vi "Table_AddNewChannelToChannelList.vi"(10 "Channel":T1, 11 "Channels":T1[](array[typedef])) -> (3 "Channels Out":T1[](array[typedef]))   [LabVIEW 2012, in "TableSupportLib.lvlib"]
uses:
  TableSupportLib.lvlib
  Table_ChannelInfoCluster.ctl
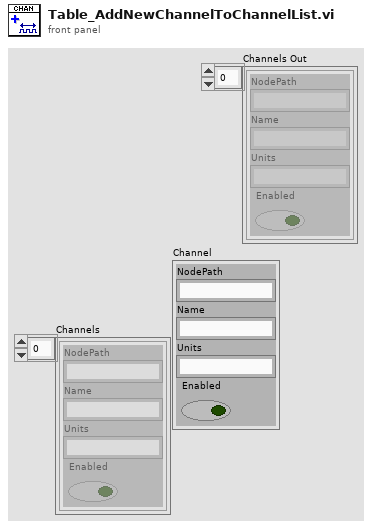
[diagram p1: front panel]
types:
  T1 = typedef "TableSupportLib.lvlib/Table_ChannelInfoCluster.ctl" = cluster{"NodePath":string, "Name":string, "Units":string, "Enabled":bool}
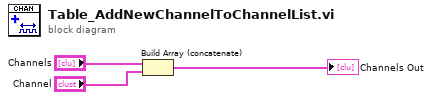
[diagram p0: block diagram]
diagram:
  n1 = Build Array (concatenate)("Channels", "Channel") -> (→"Channels Out":T1[])
